vi "Test Process Wire Branching Contains Same Data After Stopping.vi"(8 "error in (no error)":errorcluster, 11 "Process Test In":refnum<class "Process Test.lvclass">) -> (0 "error out":errorcluster, 3 "Process Test Out":refnum<class "Process Test.lvclass">)   [LabVIEW 2020, in "Process Test.lvclass"]
uses:
  Process Test.lvclass
  C:/Program Files (x86)/National Instruments/LabVIEW 2020/vi.lib/Asteme/LUnit/Test Case.lvclass
  Mock Error Handler/Mock Error Handler.lvclass
  C:/Users/anton/Documents/GitHub/Triarc-Framework/source/Framework/Error Handler Interface/Error Handler Interface.lvclass
  Framework/Process/Process.lvclass/Process.ctl
  <vilib>/Asteme/LUnit/Test Case.lvclass/Test Case.ctl
  <vilib>/Asteme/LUnit/LUnit Assertion Result.lvclass/LUnit Assertion Result.ctl
  Framework/Process/Protected/Messaging/Enqueue Message.vi
  <vilib>/Utility/error.llb/Clear Errors.vi
  Framework/Process/Private/SubVIs/Wait for finish.vi
  Framework/Process/Private/SubVIs/Set Lifecycle State.vi
  <vilib>/Asteme/LUnit/Palette/Fail.vi
  <vilib>/Asteme/LUnit/Palette/Pass.vi
  <vilib>/Asteme/LUnit/Variant to string.vi
  <vilib>/Asteme/LUnit/Set Assertion Type.vi
  <vilib>/AdvancedString/1D String Array to Delimited String.vi
  <vilib>/Asteme/LUnit/Add test result.vi
  <vilib>/Asteme/LUnit/LUnit Write Passed.vi
  <vilib>/Asteme/LUnit/LUnit Get Test Case.vi
  <vilib>/Asteme/LUnit/LUnit Write Message.vi
  <vilib>/Asteme/LUnit/LUnit Write Description.vi
  <vilib>/Asteme/LUnit/LUnit Write Assertion Type.vi
  <vilib>/Asteme/LUnit/Read Test Case Name.vi
  <vilib>/Utility/error.llb/Error Cluster From Error Code.vi
  <vilib>/Asteme/LUnit/Assertion Result/LUnit Get Test Name.vi
  <vilib>/Utility/Data Type/Get Type Information.vi
  <vilib>/Utility/LVClass/Get LV Class Name.vi
  Framework/Process/Process.lvclass
  <vilib>/Asteme/LUnit/LUnit Assertion Result.lvclass
  <vilib>/Asteme/LUnit/Test Case.lvclass
  C:/Users/anton/Documents/GitHub/Triarc-Framework/source/Framework/Base/Base.lvclass
  C:/Users/anton/Documents/GitHub/Triarc-Framework/source/Framework/Configuration File/Configuration File.lvclass
  C:/Users/anton/Documents/GitHub/Triarc-Framework/source/Framework/Process/Process.lvclass
  C:/Users/anton/Documents/GitHub/Triarc-Framework/source/Framework Test/Base Class Test/Base Class Test.lvclass
  C:/Users/anton/Documents/GitHub/Triarc-Framework/source/Framework Test/Process Test/Process Test.lvclass
  C:/Users/anton/Documents/GitHub/Triarc-Framework/source/Framework Test/Mock Error Handler/Mock Error Handler.lvclass
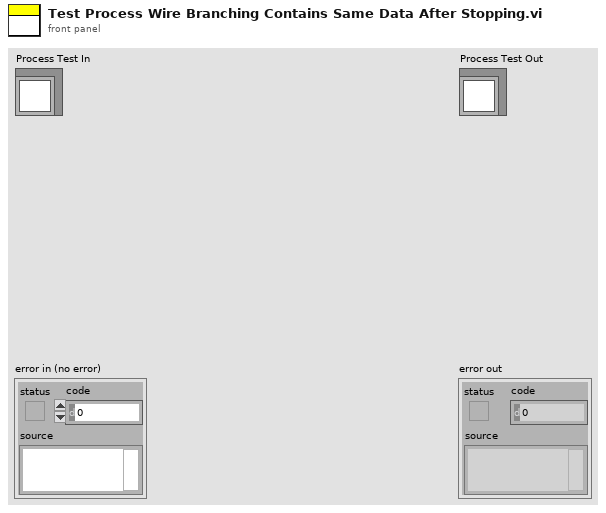
[diagram p1: front panel]
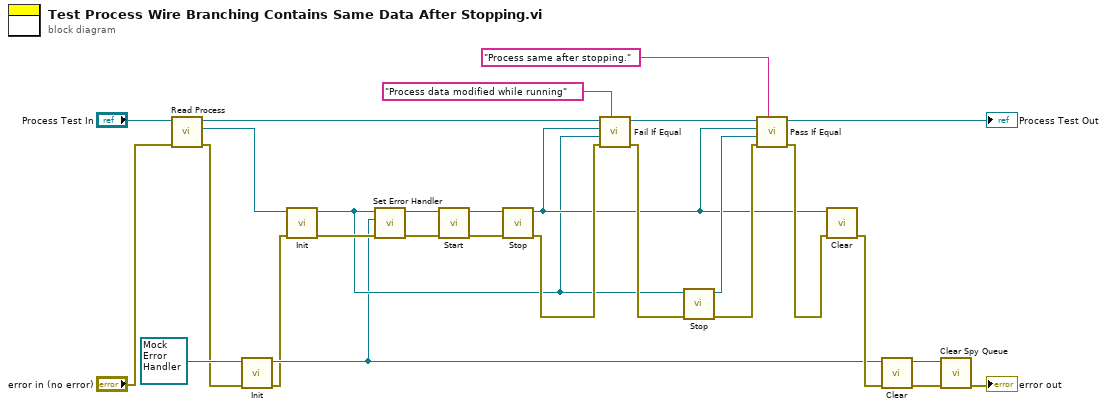
[diagram p0: block diagram]
diagram:
  n1 = call "Read Process.vi"("error in (no error)"="error in (no error)", "Process Test in"="Process Test In") -> ("error out"=w1:errorcluster, "Process.lvclass"=w22:refnum<class "Process.lvclass">, "Process Test out"=w27:refnum<class "Process Test.lvclass">)  [unwired: 7 in]
  n2 = call-dynamic "Init.vi"("error in (no error)"=w1, "Mock Error Handler In"=refnum<class "Mock Error Handler.lvclass"> refnum ("Mock Error Handler.lvclass")) -> ("error out"=w2:errorcluster, "Mock Error Handler Out"=w3:refnum<class "Mock Error Handler.lvclass">)  [unwired: 8 in]
  n3 = call-dynamic "Init.vi"("error in (no error)"=w2, "Process In"=w22) -> ("error out"=w21:errorcluster, "Process Out"=w10:refnum<class "Process.lvclass">)  [unwired: 8 in]
  n4 = call "Set Error Handler.vi"("error in (no error)"=w21, "Error Handler"=w3, "Process In"=w10) -> ("error out"=w25:errorcluster, "Process Out"=w26:refnum<class "Process.lvclass">)  [unwired: 7 in]
  n5 = call "Start.vi"("error in (no error)"=w25, "Process In"=w26) -> ("error out"=w23:errorcluster, "Process Out"=w24:refnum<class "Process.lvclass">)  [unwired: 8 in]
  n6 = call "Stop.vi"("error in (no error)"=w23, "Process In"=w24) -> ("error out"=w14:errorcluster, "Process Out"=w11:refnum<class "Process.lvclass">)  [unwired: 7 in, 1 out]
  n7 = call <vilib>:"Fail If Equal.vi"("Description"="Process data modified while running", "error in (no error)"=w14, "Actual"=w10, "Expected"=w11, "Test Case In"=w27) -> ("error out"=w13:errorcluster, "Test Case Out"=w15:refnum<class "Process Test.lvclass">)  [unwired: 5 in]
  n8 = call "Stop.vi"("error in (no error)"=w13, "Process In"=w10) -> ("error out"=w19:errorcluster, "Process Out"=w17:refnum<class "Process.lvclass">)  [unwired: 7 in, 1 out]
  n9 = call <vilib>:"Pass If Equal.vi"("Description"="Process same after stopping.", "error in (no error)"=w19, "Actual"=w17, "Expected"=w11, "Test Case In"=w15) -> ("error out"=w18:errorcluster, "Test Case Out"=→"Process Test Out":refnum<class "Process Test.lvclass">)  [unwired: 5 in]
  n10 = call-dynamic "Clear.vi"("error in (no error)"=w18, "Process In"=w11) -> ("error out"=w9:errorcluster)  [unwired: 8 in, 1 out]
  n11 = call-dynamic "Clear.vi"("error in (no error)"=w9, "Process In"=w3) -> ("error out"=w6:errorcluster, "Process Out"=w4:refnum<class "Mock Error Handler.lvclass">)  [unwired: 8 in]
  n12 = call-dynamic "Clear Spy Queue.vi"("error in (no error)"=w6, "Mock Process In"=w4) -> ("error out"=→"error out":errorcluster)  [unwired: 8 in, 1 out]
